vi "总磷氨氮插入数据.vi"(0 "table":string, 5 "data":T2={"时间标识"=timestamp(0 s since 1904-01-01), "测量模式"=enum."水样测试", "数据标记表"="N", "监测值"=0.0, "单位"=0, "数据标识"="", "因子编码"=0, "标样参考值"=0.0, "F0"=0.0, "F1"=0.0, "F2"=0.0, "F3"=0.0, "F4"=0.0, "F5"=0.0, "F6"=0.0, "F7"=0.0, "X"=0.0, "温度"=0.0, "湿度"=0.0, "量程标识"="", "SN"="", "跨度值"=0.0, "X1"=0.0} {"单位" items=["μg/L", "mg/L", "ppm", "mg/m3", "cm", "ppb", "μg/m3", "%", "nmol/mol", "μmol/mol", "MPN/L", "MPN/100ml", "ng/m3", "NTU", "无量纲", "ms/cm", "μs/cm"]}, 7 "关键参数":T1, 11 "error in (no error)":errorcluster) -> (15 "error out":errorcluster)   [LabVIEW 2016, in "斯坦道通用流路CODmn.lvlib"]
uses:
  <vilib>/Utility/error.llb/DialogType.ctl
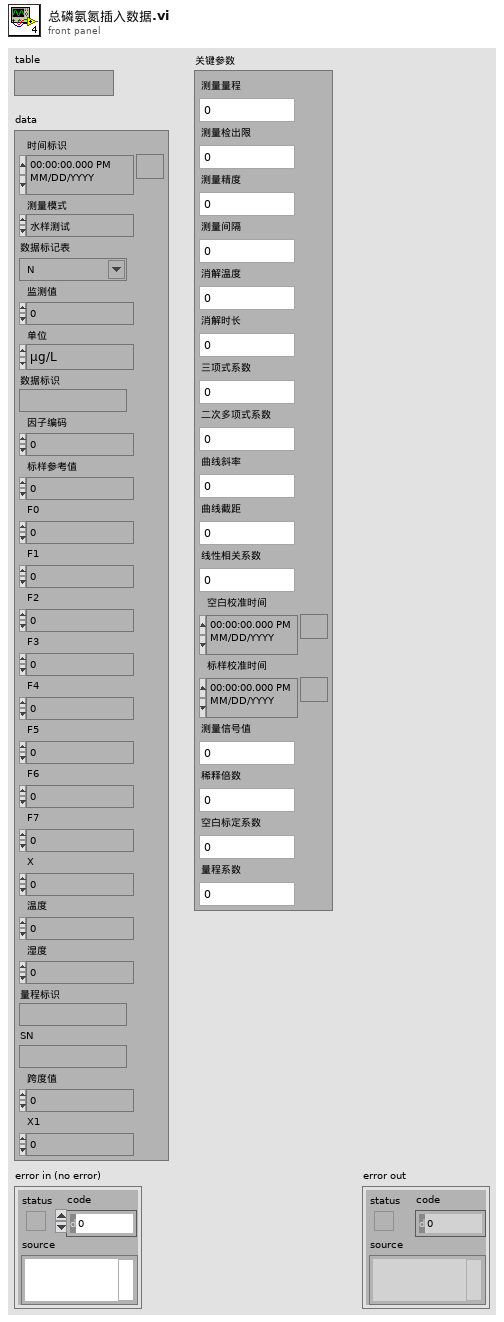
[diagram p1: front panel]
types:
  T1 = typedef "斯坦道通用流路CODmn.lvlib/关键参数.ctl" = cluster{"测量量程":sgl, "测量检出限":sgl, "测量精度":sgl, "测量间隔":sgl, "消解温度":sgl, "消解时长":sgl, "三项式系数":sgl, "二次多项式系数":sgl, "曲线斜率":sgl, "曲线截距":sgl, "线性相关系数":sgl, "空白校准时间":timestamp, "标样校准时间":timestamp, "测量信号值":sgl, "稀释倍数":sgl, "空白标定系数":sgl, "量程系数":sgl}
  T2 = cluster{"时间标识":timestamp, "测量模式":enum16{"维护数据", "水样测试", "标样核查", "零点核查", "跨度核查", "空白测试", "平行样测试", "加标回收", "空白校准", "标样校准", "初始化（清洗）", "快捷测试"}, "数据标记表":string, "监测值":sgl, "单位":u16, "数据标识":string, "因子编码":u32, "标样参考值":sgl, "F0":sgl, "F1":sgl, "F2":sgl, "F3":sgl, "F4":sgl, "F5":sgl, "F6":sgl, "F7":sgl, "X":sgl, "温度":sgl, "湿度":sgl, "量程标识":string, "SN":string, "跨度值":sgl, "X1":sgl}
  T3 = typedef "DialogType.ctl" = u16
  T4 = typedef "营养盐字段定义.ctl" = cluster{"时间":timestamp, "测量模式":string, "数据类型":string, "检测值":sgl, "单位":string, "数据标识":string, "X":sgl, "量程标识":string, "SN":string, "标样参考值":sgl, "跨度值":sgl, "F0":sgl, "F1":sgl, "F2":sgl, "F3":sgl, "F4":sgl, "F5":sgl, "F6":sgl, "F7":sgl, "X1":sgl, "因子编码":string, "温度":sgl, "湿度":sgl, "测量量程":sgl, "测量检出限":sgl, "测量精度":sgl, "测量间隔":sgl, "消解温度":sgl, "消解时长":sgl, "三项式系数":sgl, "二次多项式系数":sgl, "曲线斜率":sgl, "曲线截距":sgl, "线性相关系数":sgl, "空白校准时间":timestamp, "标样校准时间":timestamp, "测量信号值":sgl, "稀释倍数":sgl, "空白标定系数":sgl, "量程系数":sgl, "LastTime":timestamp}
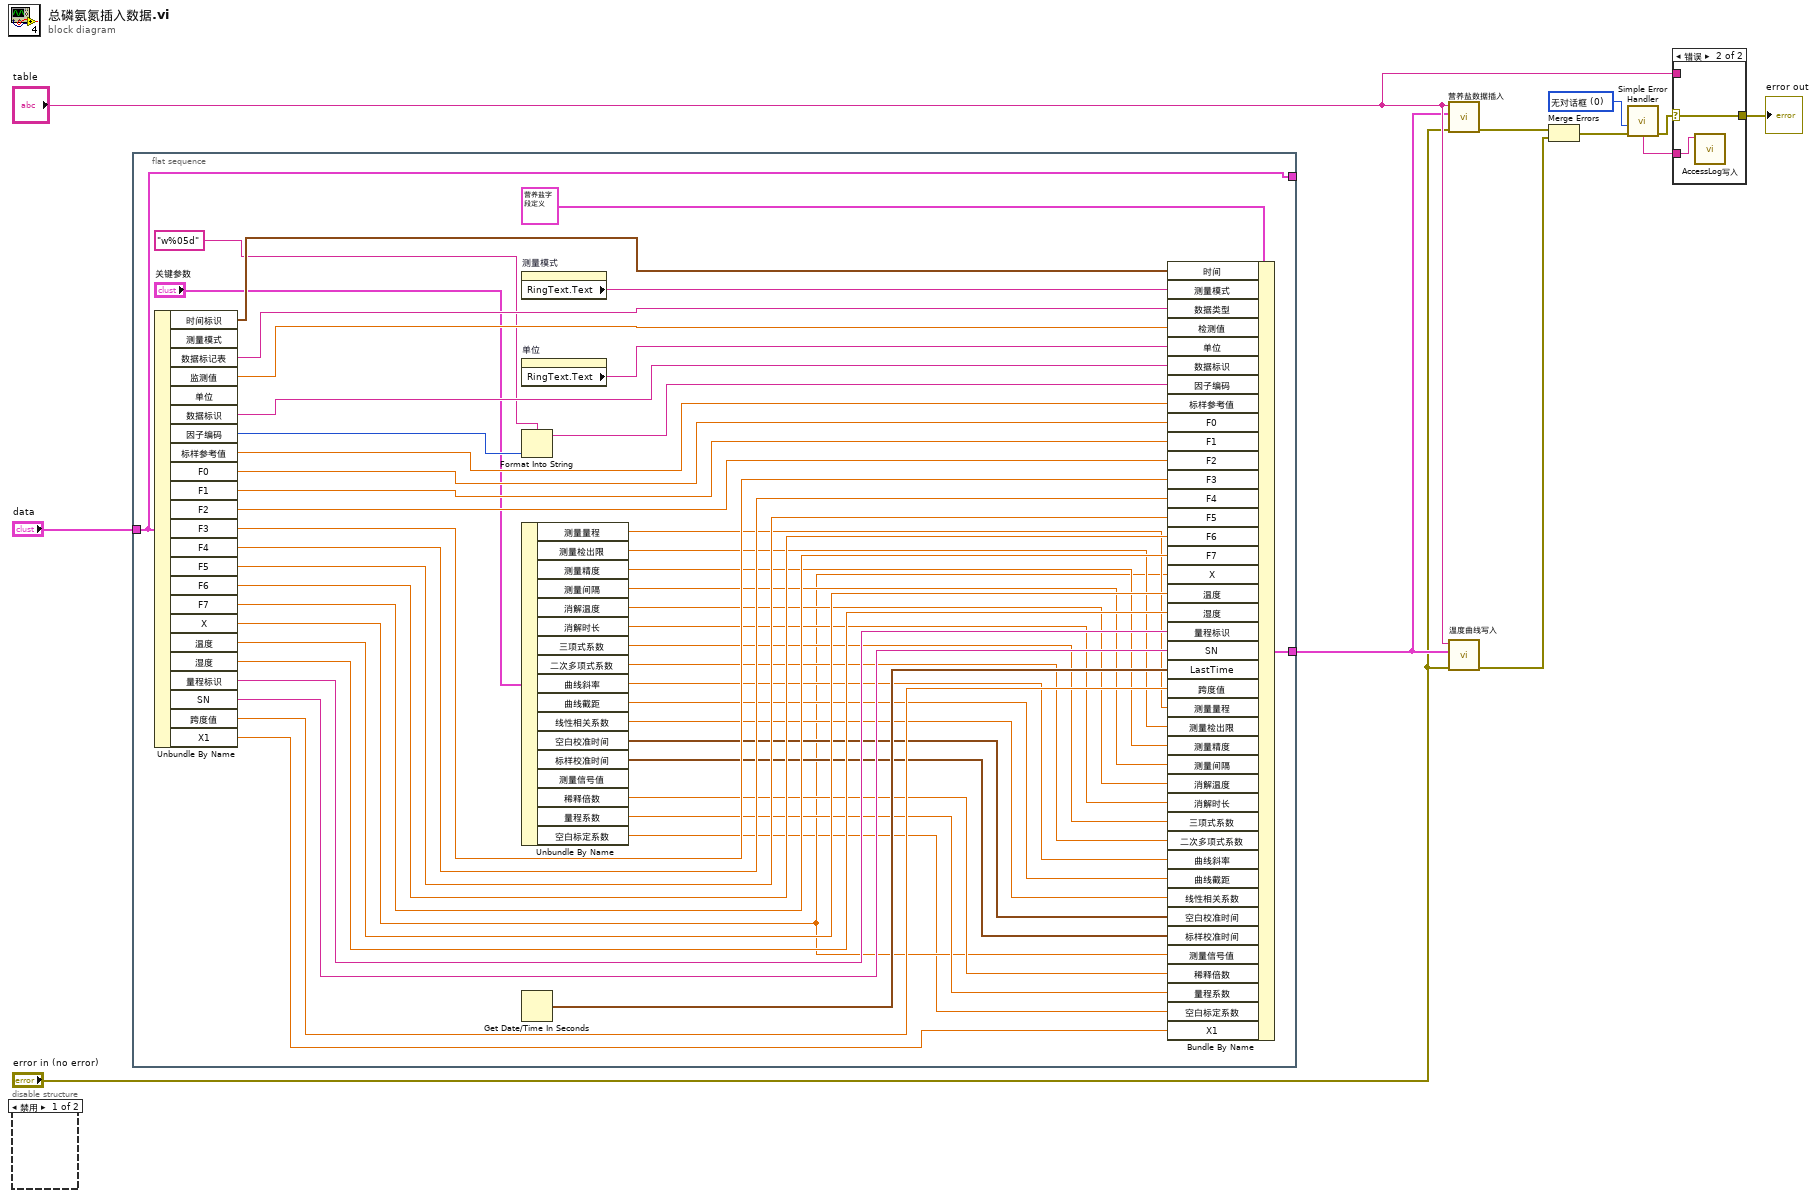
[diagram p0: block diagram]
diagram:
  w11 = T3 0 items=["无对话框", "确定信息", "继续或停止信息", "确定信息＋警告", "继续/停止+警告"] ("type of dialog (OK msg:1)")
  n1 = disable-structure shown="禁用" {
    frame Disabled {
    }
    frame Enabled {
    }
  }
  n2 = flat-sequence {
    tunnel: "data" -> [w37]
    tunnel: [w37] -> _
    tunnel: [w12] -> w4
    frame #0 {
      n3 = Unbundle By Name(w37) -> ("时间标识"=w57:timestamp, "数据标记表"=w55:string, "监测值"=w54:sgl, "数据标识"=w52:string, "因子编码"=w36:u32, "标样参考值"=w51:sgl, "F0"=w50:sgl, "F1"=w49:sgl, "F2"=w48:sgl, "F3"=w47:sgl, "F4"=w46:sgl, "F5"=w45:sgl, "F6"=w44:sgl, "F7"=w43:sgl, "X"=w16:sgl, "温度"=w42:sgl, "湿度"=w41:sgl, "量程标识"=w40:string, "SN"=w39:string, "跨度值"=w33:sgl, "X1"=w14:sgl)  [unwired: 2 out]
      n4 = property on="测量模式" class="Enum (严格)"() -> ("RingText.Text"=w56:string)  [unwired: 2 in, 2 out]
      n5 = property on="单位" class="Ring (严格)"() -> ("RingText.Text"=w53:string)  [unwired: 2 in, 2 out]
      n6 = Format Into String(format string="w%05d" ("格式字符串"), w36) -> (resulting string=w34:string)  [unwired: 2 in, 1 out]
      n7 = Unbundle By Name("关键参数") -> ("测量量程"=w31:sgl, "测量检出限"=w30:sgl, "测量精度"=w29:sgl, "测量间隔"=w28:sgl, "消解温度"=w27:sgl, "消解时长"=w26:sgl, "三项式系数"=w25:sgl, "二次多项式系数"=w24:sgl, "曲线斜率"=w23:sgl, "曲线截距"=w22:sgl, "线性相关系数"=w21:sgl, "空白校准时间"=w20:timestamp, "标样校准时间"=w19:timestamp, "稀释倍数"=w18:sgl, "量程系数"=w17:sgl, "空白标定系数"=w15:sgl)  [unwired: 1 out]
      n8 = Get Date/Time In Seconds() -> (seconds since 1Jan1904=w38:timestamp)
      n9 = Bundle By Name(cluster=T4 {"时间"=timestamp(0 s since 1904-01-01), "测量模式"="水样测试", "数据类型"="N", "检测值"=0.0, "单位"="mg/L", "数据标识"="N", "X"=0.0, "量程标识"="", "SN"="", "标样参考值"=0.0, "跨度值"=0.0, "F0"=0.0, "F1"=0.0, "F2"=0.0, "F3"=0.0, "F4"=0.0, "F5"=0.0, "F6"=0.0, "F7"=0.0, "X1"=0.0, "因子编码"="", "温度"=0.0, "湿度"=0.0, "测量量程"=0.0, "测量检出限"=0.0, "测量精度"=0.0, "测量间隔"=0.0, "消解温度"=0.0, "消解时长"=0.0, "三项式系数"=0.0, "二次多项式系数"=0.0, "曲线斜率"=0.0, "曲线截距"=0.0, "线性相关系数"=0.0, "空白校准时间"=timestamp(0 s since 1904-01-01), "标样校准时间"=timestamp(0 s since 1904-01-01), "测量信号值"=0.0, "稀释倍数"=0.0, "空白标定系数"=0.0, "量程系数"=0.0, "LastTime"=timestamp(0 s since 1904-01-01)} ("data"), "时间"=w57, "测量模式"=w56, "数据类型"=w55, "检测值"=w54, "单位"=w53, "数据标识"=w52, "因子编码"=w34, "标样参考值"=w51, "F0"=w50, "F1"=w49, "F2"=w48, "F3"=w47, "F4"=w46, "F5"=w45, "F6"=w44, "F7"=w43, "X"=w16, "温度"=w42, "湿度"=w41, "量程标识"=w40, "SN"=w39, "LastTime"=w38, "跨度值"=w33, "测量量程"=w31, "测量检出限"=w30, "测量精度"=w29, "测量间隔"=w28, "消解温度"=w27, "消解时长"=w26, "三项式系数"=w25, "二次多项式系数"=w24, "曲线斜率"=w23, "曲线截距"=w22, "线性相关系数"=w21, "空白校准时间"=w20, "标样校准时间"=w19, "测量信号值"=w16, "稀释倍数"=w18, "量程系数"=w17, "空白标定系数"=w15, "X1"=w14) -> (w12:T4)
    }
  }
  n10 = call "营养盐数据插入.vi"("Tabe Name"="table", "data"=w4, "错误输入（无错误）"="error in (no error)") -> ("错误输出"=w6:errorcluster)  [unwired: 7 in]
  n11 = call "温度曲线写入.vi"("error in (no error)"="error in (no error)", "columns"=w4, "table"="table") -> ("错误输出"=w1:errorcluster)  [unwired: 8 in]
  n12 = Merge Errors(w6, w1) -> (w2:errorcluster)
  n13 = call <vilib>:"Simple Error Handler.vi"("type of dialog (OK msg:1)"=w11, "error in (no error)"=w2) -> ("error out"=w10:errorcluster, "message"=w9:string)  [unwired: 3 in, 3 out]
  n14 = case shown="错误" w10 {
    selector: w10 -> [_ w58]
    tunnel: w9 -> [_ w59]
    tunnel: [_ w58] -> w8
    tunnel: "table" -> [_ _]
    frame No Error {
    }
    frame Error {
      n15 = call "AccessLog写入.vi"("Log"=w59) -> ()  [unwired: 11 in]
    }
  }
  "error out" <- w8
